vi "R2FIR.vi"(1 "Parity":enum16{"Odd", "Even"}(ring), 2 "Frequency":dbl[](array[numeric]), 4 "Phase":dbl[](array[numeric])) -> (5 "FIR coefficients":dbl[](array[numeric]))   [LabVIEW 2018]
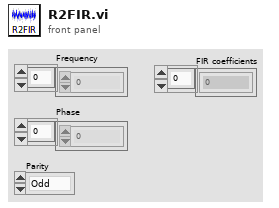
[diagram p1: front panel]
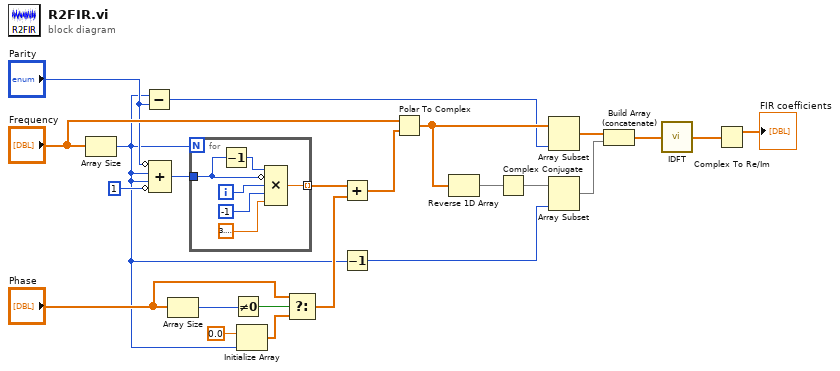
[diagram p0: block diagram]
diagram:
  n1 = Array Size(array="Frequency") -> (size(s)=w1:i32)
  n2 = Subtract(x=w1, y="Parity") -> (x-y=w17:i32)
  n3 = Compound Arithmetic op=ADD(invert "Parity", w1, w1, invert 1) -> (w23:i32)
  n4 = Array Size(array="Phase") -> (size(s)=w4:i32)
  n5 = for {
    N: w1 -> [_]
    tunnel: [w28] -> w9 mode=indexing
    tunnel: w23 -> [w24]
    i -> [w27]
    n6 = Decrement(x=w24) -> (x-1=w29:i32)
    n7 = Compound Arithmetic op=MULTIPLY(w29, invert w24, w27, -1 ("value"), 3.141592653589793) -> (w28:dbl)
  }
  n8 = Not Equal To 0?(x=w4) -> (x != 0?=w7:bool)
  n9 = Initialize Array(0.0 ("element"), w1) -> (w6:dbl[])
  n10 = Select(t="Phase", s=w7, f=w6) -> (s? t:f=w3:dbl[])
  n11 = Add(x=w9, y=w3) -> (x+y=w8:dbl[])
  n12 = Decrement(x=w1) -> (x-1=w15:i32)
  n13 = Polar To Complex(1:w8, 2:"Frequency") -> (0:w19:cdb[])
  n14 = Reverse 1D Array(array=w19) -> (reversed array=w20:cdb[])
  n15 = Complex Conjugate(1:w20) -> (0:w16:cdb[])
  n16 = Array Subset(array=w19, length=w17) -> (w14:cdb[])  [unwired: 1 in]
  n17 = Array Subset(array=w16, length=w15) -> (w13:cdb[])  [unwired: 1 in]
  n18 = Build Array (concatenate)(w14, w13) -> (w12:cdb[])
  n19 = call "IDFT.vi"("Input"=w12) -> ("Output"=w11:cdb[])
  n20 = Complex To Re/Im(x + iy=w11) -> (x=→"FIR coefficients":dbl[])  [unwired: 1 out]
